vi "SJ_Stats.vi"() -> (5 "Plug in titles":string[](array[string])=["SJ:Characteristic:Velocity", "SJ:Velocity:Phase_Angle"], 7 "Plug in values":string[](array[string])=["4.470676", "-87.866783"])   [LabVIEW 2011]
uses:
  Globals/Meas_global.vi
  <vilib>/Analysis/2dsp.llb/1D Cross Correlation (DBL).vi
  <vilib>/Analysis/1siggen.llb/Ramp Pattern by Delta.vi
  <vilib>/Analysis/NI_AALBase.lvlib
  <vilib>/Analysis/NI_AAL_SigProc.lvlib
  <vilib>/Analysis/NI_AALPro.lvlib
panel:
  out "Signal Time Lag":dbl
  in  "Jet Frequency":dbl=950.0
  out "Peak Velocity":dbl
  out "Characteristic Velocity":dbl
  out "Velocity Threshold":dbl
  out "Jet Phase Angle":dbl
  in  "Voltage Name":string="RV (Vin)"
  in  "Velocity Name":string="HW (Uhw)"
  out "SJ Velocity":cluster{"Ramp Pattern":dbl[], dbl[]}[](graph)
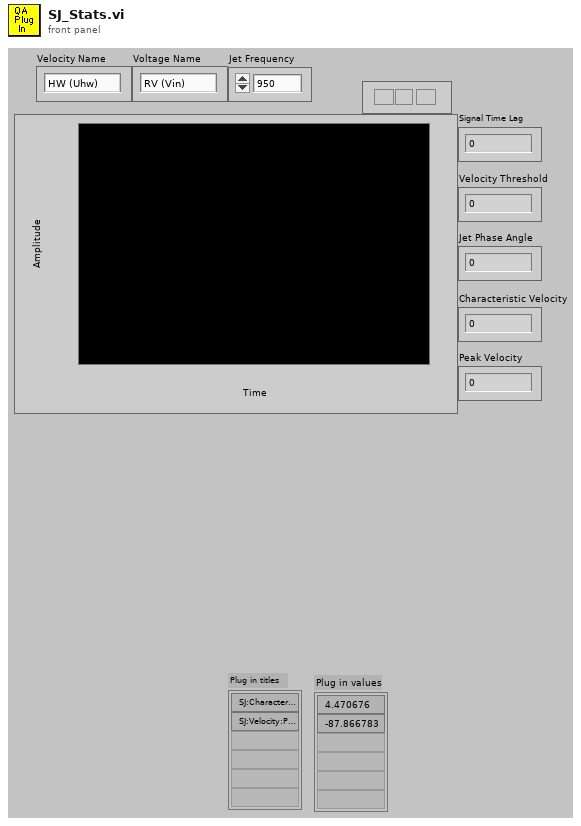
[diagram p1: front panel]
types:
  T1 = typedef "Analysis_info_cluster.ctl" = cluster{"Colour":u32, "Inst type":T2, "Inst name":string, "Symbol":string, "Code name":string, "Extra Info":string, "Inst Array":T3, "Extra Titles":string[], "Extra Values":string[], "Eng Values":dbl[], "Time (ms)":dbl[], "Voltage":dbl[], "U":dbl, "u^2":dbl, "u^3":dbl, "u^4":dbl, "Skew_u":dbl, "Kurt_u":dbl, "Sd Error in Mean":dbl, "% u'/U":dbl, "X":dbl, "Y":dbl, "Z":dbl, "Spectra":T4, "Autocorrelation":T4, "Timescale integral to 25%":dbl, "Sd Error in Variance":dbl, "Calib File":path, "Calib Constants":dbl[], "Histogram":T4, "Output Position":bool, "Full Stats":bool, "Weighting":dbl[], "Av Sampling Rate":dbl, "Av No of Samples":dbl, "Total Meas Time (s)":dbl}
  T2 = typedef "Inst_type.ctl" = enum16{"Propeller anemometer", "Raw voltage", "Pressure Transducer", "Pitot-static tube", "Preston tube", "Hot wire", "Cross wire 1", "Cross wire 2", "Generic Linear", "Generic Polynomial", "Generic BackPoly", "Fast FID", "Thermocouple", "Cold wire", "Pulsed Wire", "LDA Vel", "LDA Tran time", "LDA Arr time"}
  T3 = typedef "Instrument_Array.ctl" = enum16{"PWA", "LDA", "Analogue"}
  T4 = typedef "XY_Plot_Cluster.ctl" = cluster{"First Name":string, "Second Name":string, "X axis name":string, "Y axis name":string, "X array":dbl[], "Y array":dbl[]}
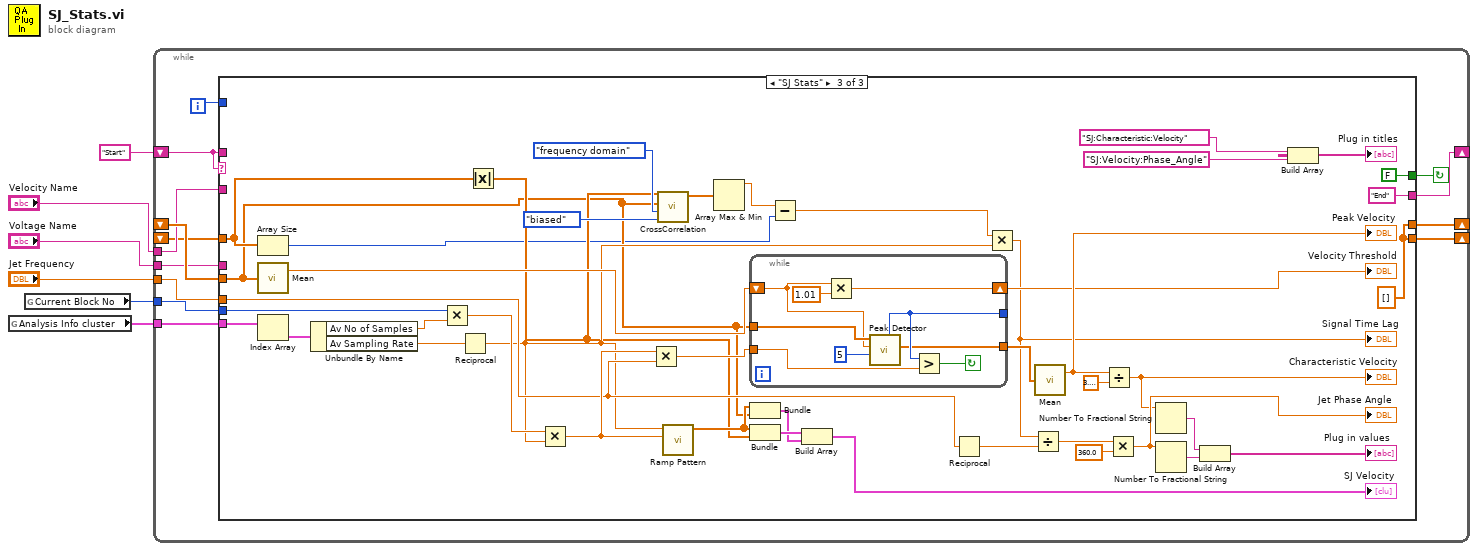
[diagram p0: block diagram]
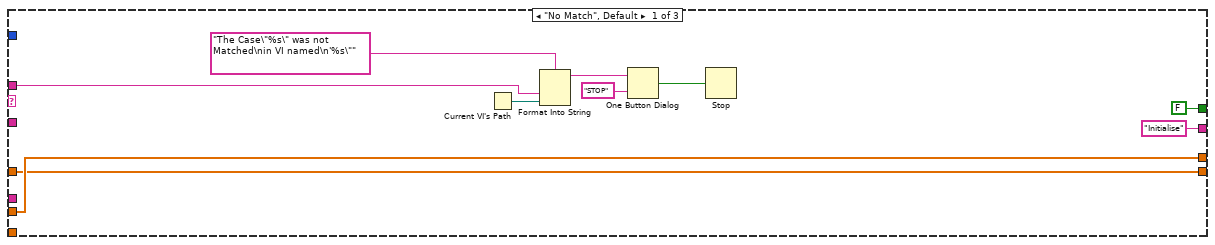
[diagram p2: hidden frame]
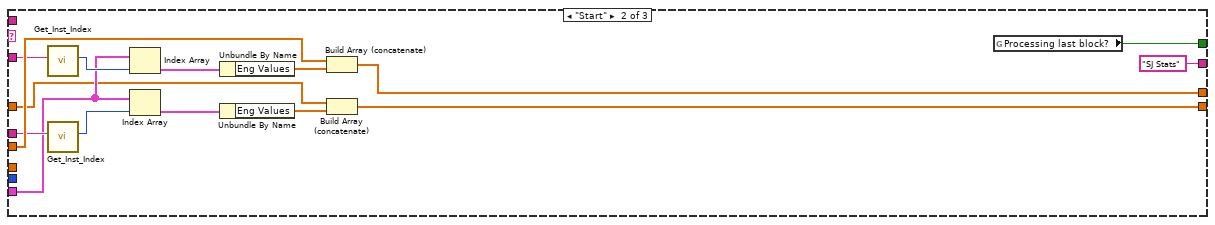
[diagram p3: hidden frame]
diagram:
  n1 = global read "Meas_global.vi" "Analysis Info cluster"() -> (w5:T1[])
  n2 = global read "Meas_global.vi" "Current Block No"() -> (w4:i32)
  n3 = while {
    shift-left: "Start" -> [w17]
    shift-right: [w18] -> _
    tunnel: w5 -> [w16]
    tunnel: w4 -> [w15]
    shift-right: [w12] -> _
    shift-left: _ -> [w13]
    tunnel: "Voltage Name" -> [w11]
    tunnel: "Velocity Name" -> [w10]
    shift-right: [w9] -> _
    shift-left: _ -> [w8]
    tunnel: "Jet Frequency" -> [w7]
    i -> [w14]
    stop <- w19 continue-if-true
    n4 = case shown="\"SJ Stats\"" w17 {
      tunnel: [FALSE w44 FALSE ("Processing last block?")] -> w19
      tunnel: ["Initialise" "SJ Stats" "End"] -> w18
      tunnel: w17 -> [w24 _ _]
      tunnel: w16 -> [_ w35 w84]
      tunnel: w15 -> [_ _ w83]
      tunnel: w14 -> [_ _ _]
      tunnel: [w21 w41 w71] -> w12
      tunnel: w13 -> [w21 w42 w48]
      tunnel: w11 -> [_ w39 _]
      tunnel: w10 -> [_ w38 _]
      tunnel: [w20 w34 w71] -> w9
      tunnel: w8 -> [w20 w33 w65]
      tunnel: w7 -> [_ _ w53]
      frame "No Match", Default {
        n5 = Current VI's Path() -> (path=w23:path)
        n6 = Format Into String(format string="The Case\"%s\" was not Matched\nin VI named\n'%s\"" ("Format String"), w24, w23) -> (resulting string=w27:string)  [unwired: 2 in, 1 out]
        n7 = One Button Dialog(message=w27, button name ("OK")="STOP") -> (true=w25:bool)
        n8 = Stop(stop? (T)=w25) -> ()
      }
      frame "Start" {
        n9 = call "Get_Inst_Index.vi"("Inst name search"=w38) -> ("Index of Instance"=w36:i32)  [unwired: 8 in, 2 out]
        n10 = call "Get_Inst_Index.vi"("Inst name search"=w39) -> ("Index of Instance"=w37:i32)  [unwired: 8 in, 2 out]
        n11 = Index Array(array=w35, index=w36) -> (element=w32:T1)
        n12 = Index Array(array=w35, index=w37) -> (element=w31:T1)
        n13 = Unbundle By Name(w32) -> ("Eng Values"=w40:dbl[])
        n14 = Unbundle By Name(w31) -> ("Eng Values"=w30:dbl[])
        n15 = Build Array (concatenate)(w42, w40) -> (w41:dbl[])
        n16 = Build Array (concatenate)(w33, w30) -> (w34:dbl[])
        n17 = global read "Meas_global.vi" "Processing last block?"() -> (w44:bool)
      }
      frame "SJ Stats" {
        w71 = dbl[] []
        n18 = Array Size(array=w65) -> (size(s)=w47:i32)
        n19 = call <vilib>:"Mean.vi"("X"=w48) -> ("mean"=w77:dbl)  [unwired: 1 out]
        n20 = Index Array(array=w84) -> (element=w85:T1)  [unwired: 1 in]
        n21 = Unbundle By Name(w85) -> ("Av No of Samples"=w72:dbl, "Av Sampling Rate"=w73:dbl)
        n22 = Multiply(x=w83, y=w72) -> (x*y=w82:dbl)
        n23 = Reciprocal(x=w73) -> (1/x=w50:dbl)
        n24 = Absolute Value(x=w65) -> (abs(x)=w49:dbl[])
        n25 = Multiply(x=w82, y=w50) -> (x*y=w76:dbl)
        n26 = Multiply(x=w76, y=w53) -> (x*y=w63:dbl)
        n27 = call-poly <vilib>:"CrossCorrelation.vi"("normalization"=enum32{"none", "unbiased", "biased"}."biased", "algorithm"=enum32{"direct", "frequency domain"}."frequency domain", "Y"=w48, "X"=w49) -> ("Rxy"=w46:dbl[])  [unwired: 6 in, 1 out]
        n28 = call-poly <vilib>:"Ramp Pattern.vi"("end"=w76, "delta"=w50) -> ("Ramp Pattern"=w66:dbl[])  [unwired: 7 in, 2 out]
        n29 = Array Max & Min(array=w46) -> (max value=w45:dbl)  [unwired: 3 out]
        n30 = while {
          tunnel: [w95] -> _
          tunnel: w63 -> [w94]
          tunnel: w48 -> [w96]
          shift-right: [w89] -> w55
          shift-left: w77 -> [w91]
          tunnel: [w93] -> w74
          stop <- w92 continue-if-true
          n31 = Multiply(x=w91, y=1.01) -> (x*y=w89:dbl)
          n32 = call <vilib>:"Peak Detector.vi"("width"=5, "threshold"=w91, "X"=w96) -> ("Amplitudes"=w93:dbl[], "# found"=w95:i32)  [unwired: 4 in, 3 out]
          n33 = Greater?(x=w95, y=w94) -> (0:w92:bool)
        }
        "Velocity Threshold" <- w55
        n34 = Bundle("Ramp Pattern"=w66, w48) -> (w67:cluster{"Ramp Pattern":dbl[], dbl[]})  [unwired: 1 in]
        n35 = Bundle("Ramp Pattern"=w66, w49) -> (w68:cluster{"Ramp Pattern":dbl[], dbl[]})  [unwired: 1 in]
        n36 = Subtract(x=w45, y=w47) -> (x-y=w54:dbl)
        n37 = Build Array(w68, w67) -> (→"SJ Velocity":cluster{"Ramp Pattern":dbl[], dbl[]}[])
        n38 = Reciprocal(x=w53) -> (1/x=w52:dbl)
        n39 = Multiply(x=w54, y=w50) -> (x*y=w51:dbl)
        "Signal Time Lag" <- w51
        n40 = Divide(x=w51, y=w52) -> (x/y=w62:dbl)
        n41 = call <vilib>:"Mean.vi"("X"=w74) -> ("mean"=w58:dbl)  [unwired: 1 out]
        "Peak Velocity" <- w58
        n42 = Divide(x=w58, y=3.141592653589793) -> (x/y=w56:dbl)
        "Characteristic Velocity" <- w56
        n43 = Multiply(x=w62, y=360.0) -> (x*y=w57:dbl)
        "Jet Phase Angle" <- w57
        n44 = Number To Fractional String(number=w56) -> (F-format string=w78:string)  [unwired: 3 in]
        n45 = Number To Fractional String(number=w57) -> (F-format string=w59:string)  [unwired: 3 in]
        n46 = Build Array(w78, w59) -> (→"Plug in values":string[])
        n47 = Build Array("SJ:Characteristic:Velocity", "SJ:Velocity:Phase_Angle") -> (→"Plug in titles":string[])
      }
    }
  }
